vi "insertHTBinData1.vi"(8 "error in (no error)":errorcluster, 9 "FileName":string, 10 "String":string, 11 "connection reference":T2) -> (0 "error out":errorcluster, 1 "concatenated string":string, 3 "connection reference out":T2)   [LabVIEW 2012]
uses:
  <vilib>/addons/database/Connection.llb/Conn ObjectReference.ctl
  <vilib>/addons/database/NI_Database_API.lvlib
panel:
  out "output cluster 2":T1
  out "String 4":string
  out "String 3":string
  out "String 2":string
  out "substring 4":string
  out "before substring":string
  out "substring 3":string
  out "offset past match":i32
  out "after substring 3":string
  in  "input cluster  2":T1
  out "size(s)":i32
  out "E2":i32
  out "S4":string
  out "S5":string
  out "S6":string
  out "S3":string
  out "S2":string
  out "S1":string
  out "array":string[][](array[string])
  out "String":string
  out "output cluster":T1
  in  "input cluster":T1
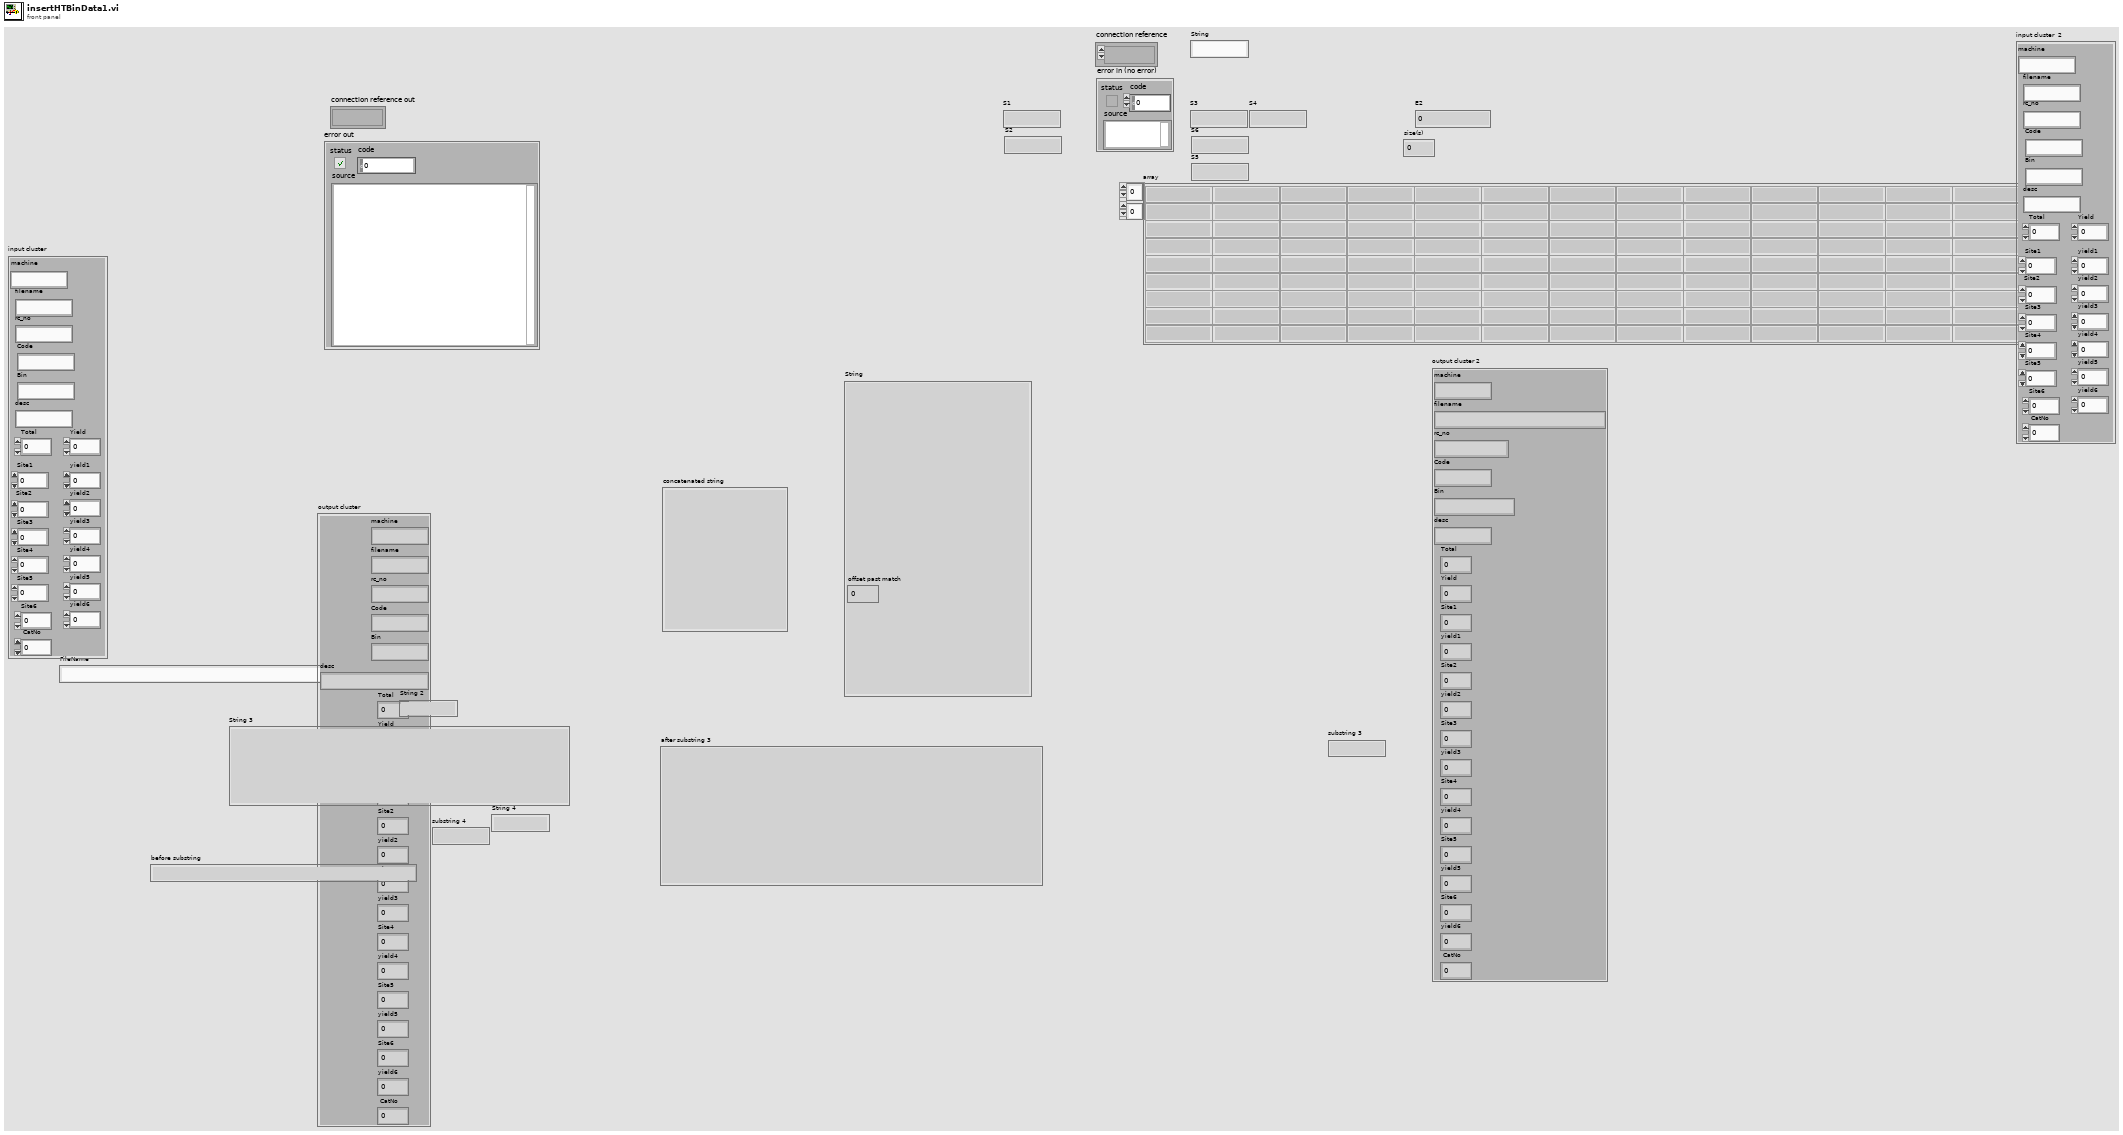
[diagram p1: front panel]
types:
  T1 = cluster{"machine":string, "filename":string, "rc_no":string, "Code":string, "Bin":string, "desc":string, "Total":dbl, "Yield":dbl, "Site1":dbl, "yield1":dbl, "Site2":dbl, "yield2":dbl, "Site3":dbl, "yield3":dbl, "Site4":dbl, "yield4":dbl, "Site5":dbl, "yield5":dbl, "Site6":dbl, "yield6":dbl, " CatNo":dbl}
  T2 = typedef "NI_Database_API.lvlib/Conn ObjectReference.ctl" = refnum<k1>
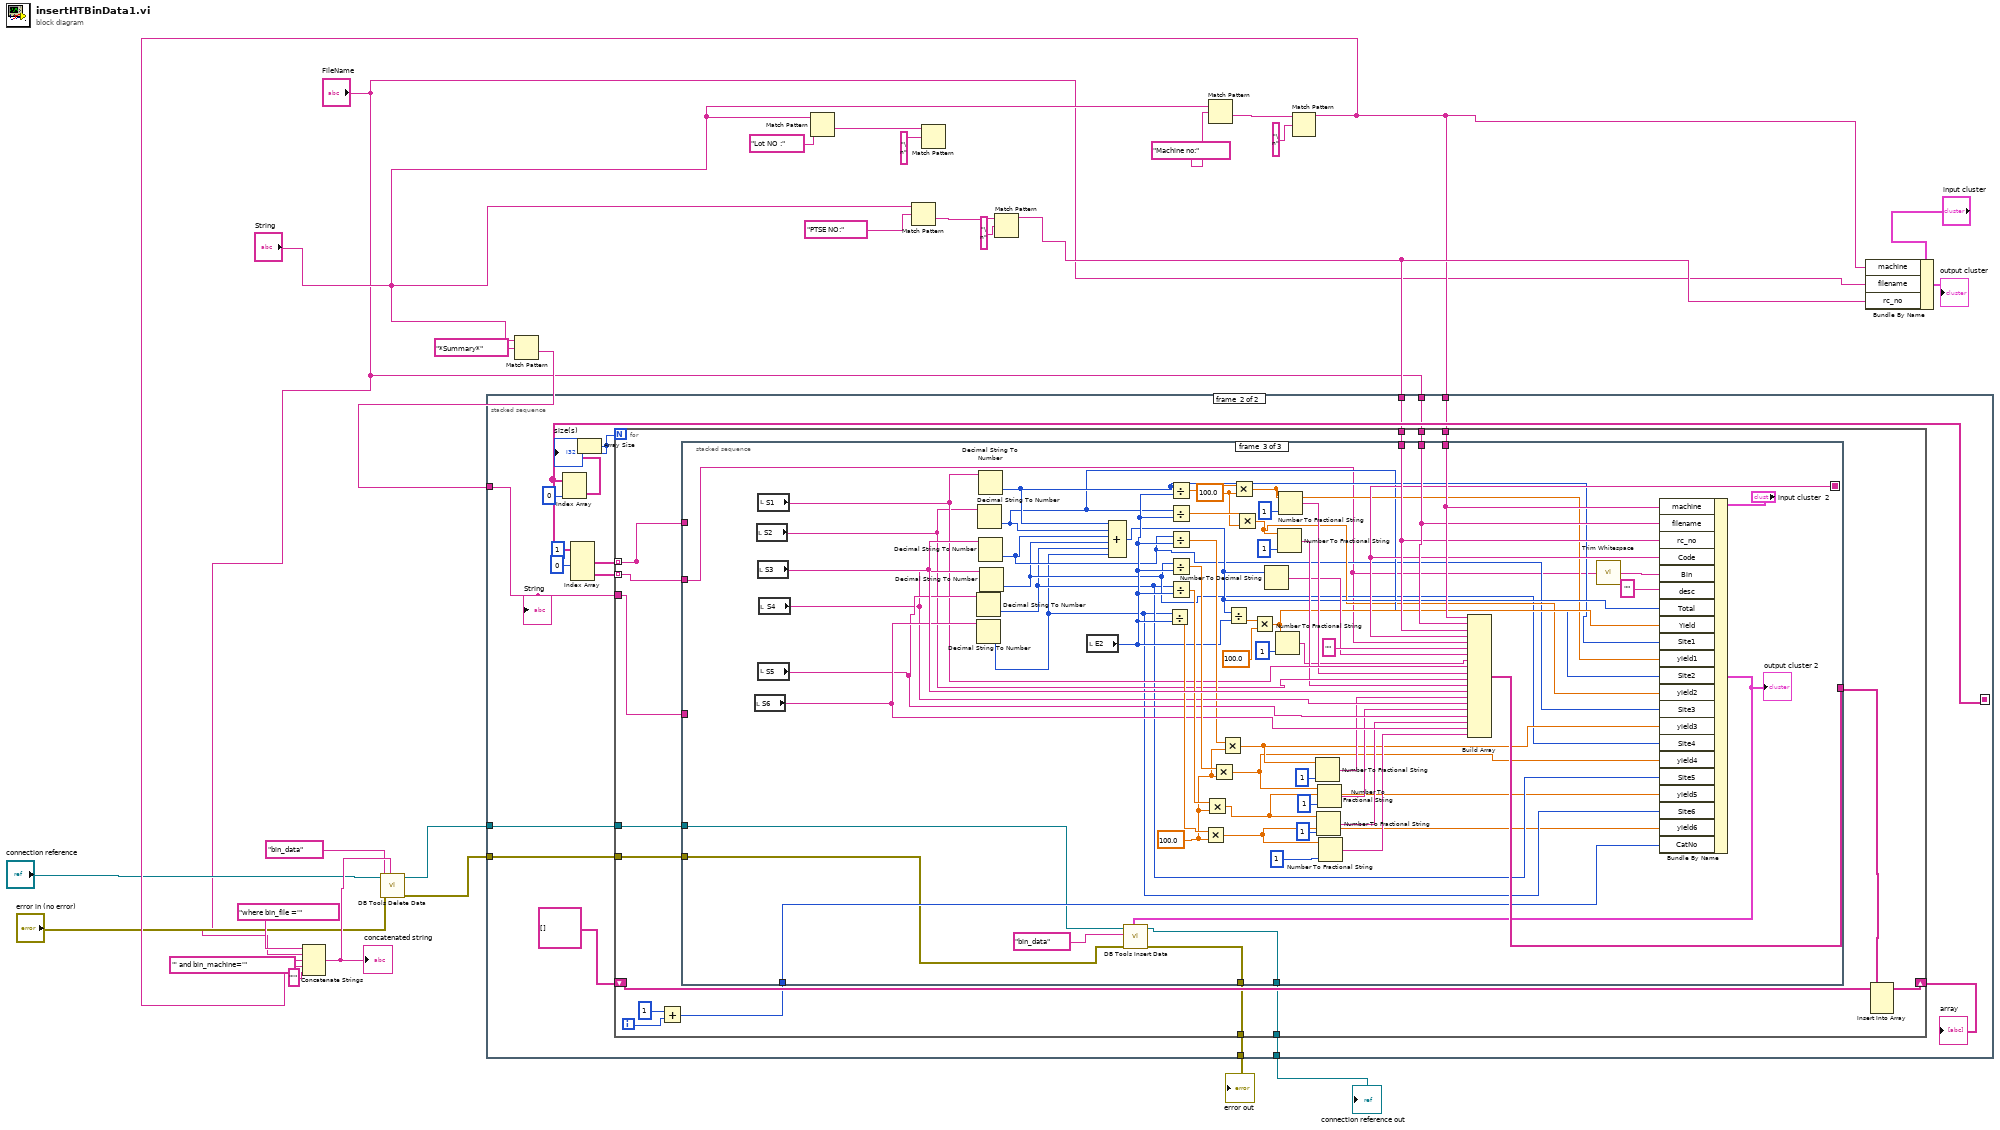
[diagram p0: block diagram]
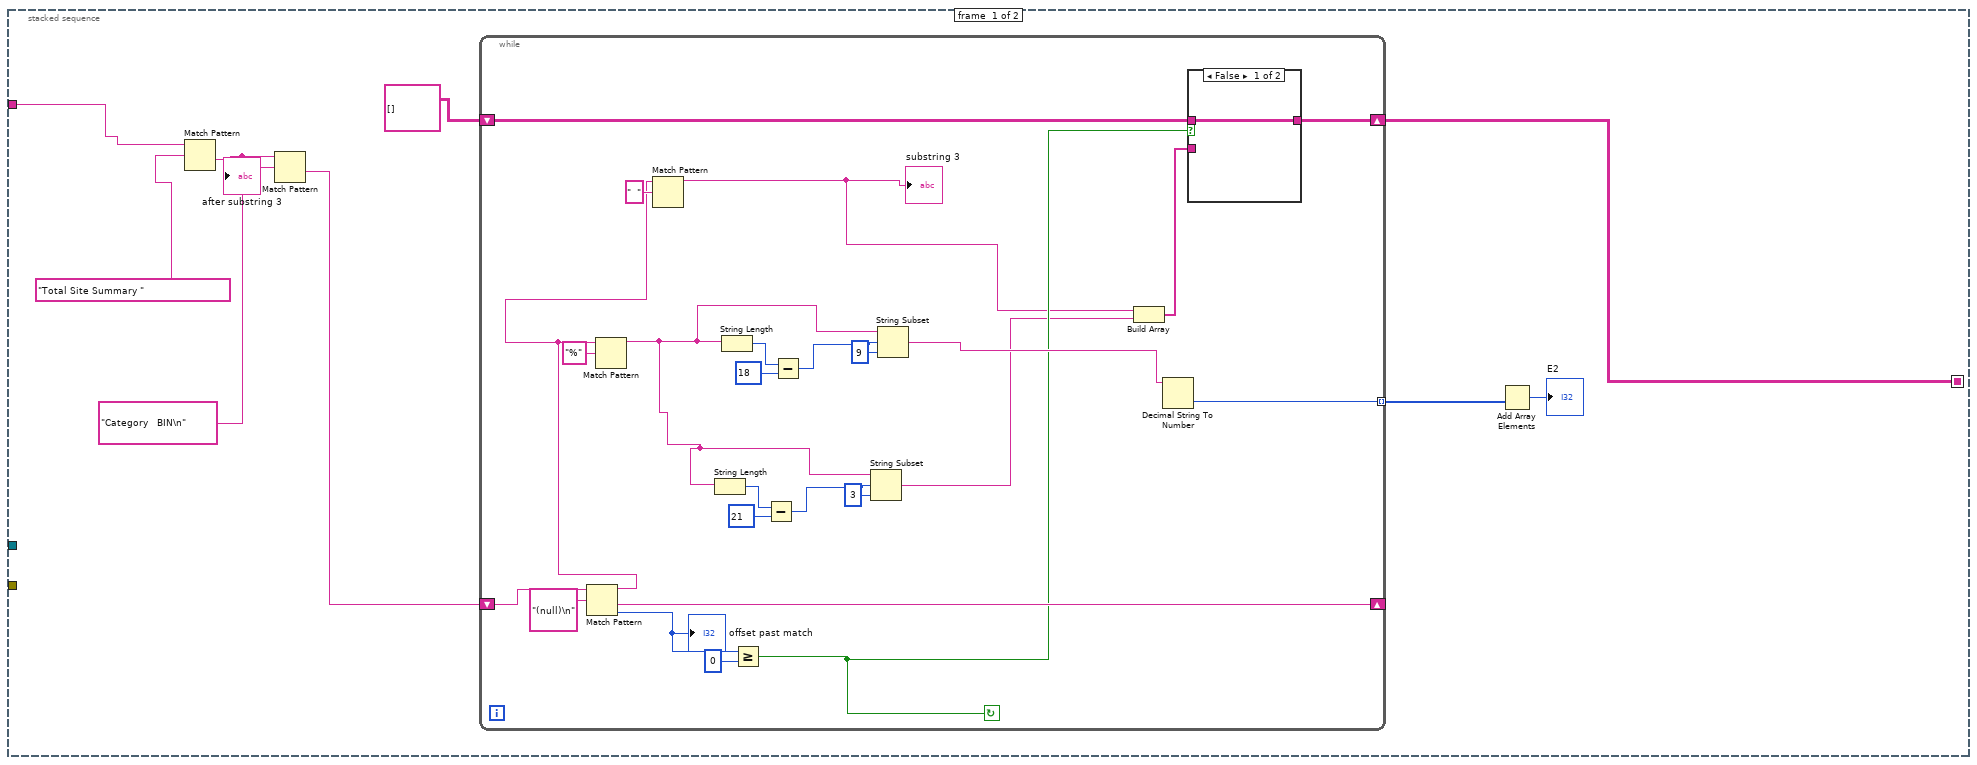
[diagram p2: hidden frame]
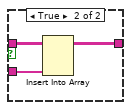
[diagram p3: hidden frame]
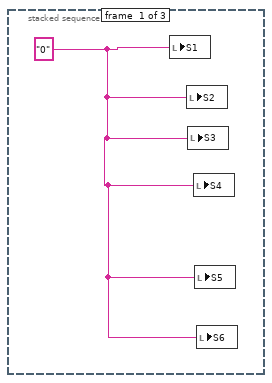
[diagram p4: hidden frame]
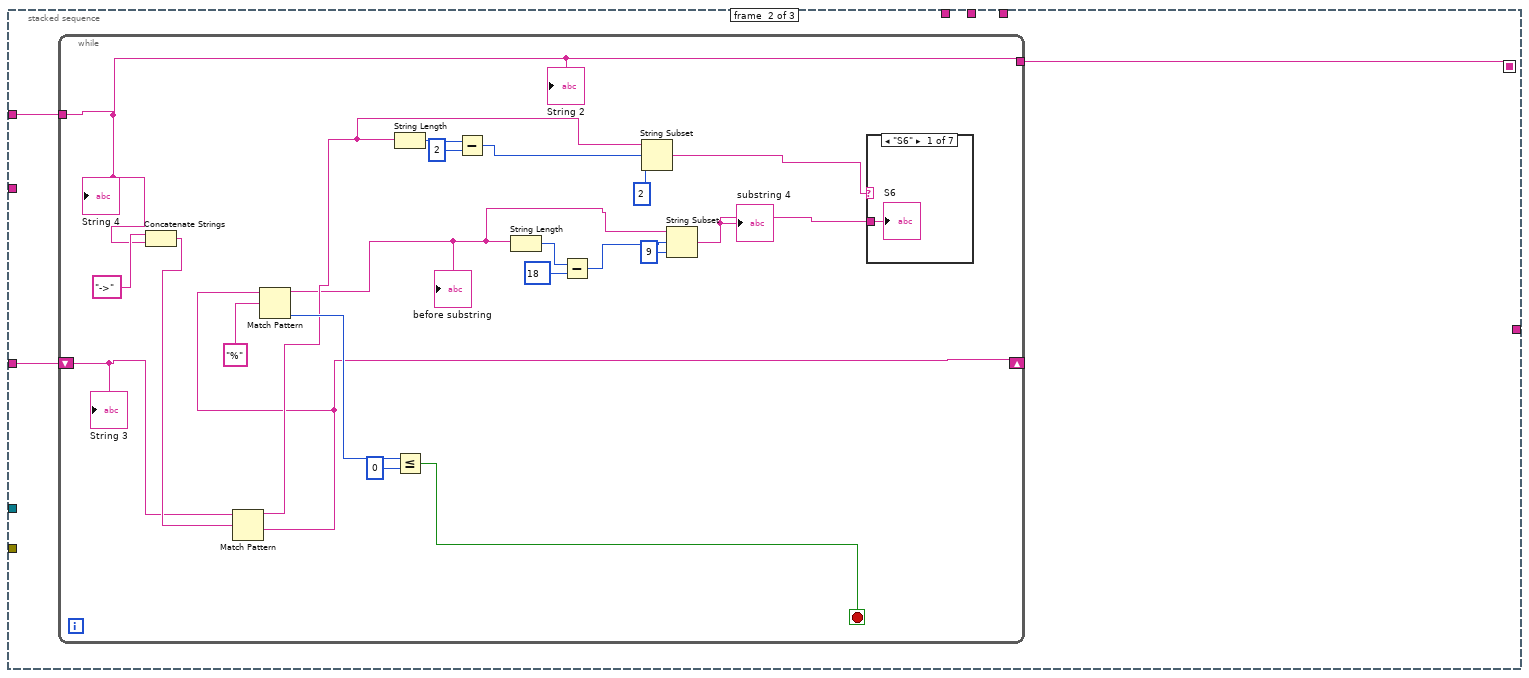
[diagram p5: hidden frame]
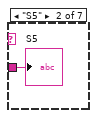
[diagram p6: hidden frame]
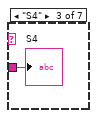
[diagram p7: hidden frame]
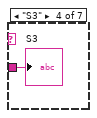
[diagram p8: hidden frame]
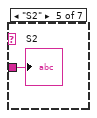
[diagram p9: hidden frame]
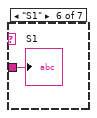
[diagram p10: hidden frame]
diagram:
  n1 = Match Pattern(string="String", regular expression="*Summary*") -> (after substring=w16:string)  [unwired: 1 in, 3 out]
  n2 = Match Pattern(string="String", regular expression="Lot NO :") -> (after substring=w27:string)  [unwired: 1 in, 3 out]
  n3 = Match Pattern(string="String", regular expression="PTSE NO:") -> (after substring=w21:string)  [unwired: 1 in, 3 out]
  n4 = Match Pattern(string=w27, regular expression="\n") -> ()  [unwired: 1 in, 4 out]
  n5 = Match Pattern(string=w21, regular expression="\n") -> (before substring=w15:string)  [unwired: 1 in, 3 out]
  n6 = Match Pattern(string="String", regular expression="Machine no:") -> (after substring=w24:string)  [unwired: 1 in, 3 out]
  n7 = Match Pattern(string=w24, regular expression="\n") -> (before substring=w9:string)  [unwired: 1 in, 3 out]
  n8 = Concatenate Strings("where bin_file ='" ("SQL query"), "FileName", "' and bin_machine='" ("string"), w9, "'" ("string")) -> (w11:string)
  "concatenated string" <- w11
  n9 = call <vilib>:"DB Tools Delete Data.vi"("condition"=w11, "error in (no error)"="error in (no error)", "table"="bin_data", "connection reference"="connection reference") -> ("error out"=w7:errorcluster, "connection reference out"=w8:T2)  [unwired: 6 in]
  n10 = stacked-sequence {
    seq-local: [w29 _] -> [_ w79]
    tunnel: w16 -> [w33 w84]
    tunnel: "FileName" -> [_ w73]
    tunnel: w9 -> [_ w72]
    tunnel: w15 -> [_ w71]
    tunnel: w8 -> [_ w70]
    tunnel: w7 -> [_ w69]
    tunnel: [_ w68] -> w2
    tunnel: [_ w67] -> w1
    frame #0 {
      n11 = Match Pattern(string=w33, regular expression="Total Site Summary ") -> (after substring=w36:string)  [unwired: 1 in, 3 out]
      "after substring 3" <- w36
      n12 = Match Pattern(string=w36, regular expression="Category   BIN\n") -> (after substring=w31:string)  [unwired: 1 in, 3 out]
      n13 = while {
        shift-right: [w50] -> _
        shift-left: w31 -> [w49]
        tunnel: [w44] -> w30 mode=indexing
        shift-right: [w42] -> w29
        shift-left: string[][] [] ("array") -> [w41]
        stop <- w40 continue-if-true
        n14 = Match Pattern(string=w49, regular expression="(null)\n") -> (before substring=w46:string, after substring=w50:string, offset past match=w48:i32)  [unwired: 1 in, 1 out]
        "offset past match" <- w48
        n15 = Match Pattern(string=w46, regular expression="%") -> (before substring=w53:string)  [unwired: 1 in, 3 out]
        n16 = Match Pattern(string=w46, regular expression="  ") -> (before substring=w39:string)  [unwired: 1 in, 3 out]
        "substring 3" <- w39
        n17 = String Length(string=w53) -> (length=w57:i32)
        n18 = String Length(string=w53) -> (length=w61:i32)
        n19 = Greater Or Equal?(x=w48, y=0) -> (x >= y?=w40:bool)
        n20 = Subtract(x=w57, y=21) -> (x-y=w55:i32)
        n21 = Subtract(x=w61, y=18) -> (x-y=w59:i32)
        n22 = String Subset(string=w53, offset (0)=w55, length (rest)=3 ("length (rest)")) -> (substring=w38:string)
        n23 = String Subset(string=w53, offset (0)=w59, length (rest)=9 ("length (rest)")) -> (substring=w45:string)
        n24 = Build Array(w39, w38) -> (w43:string[])
        n25 = Decimal String To Number(string=w45) -> (number=w44:i32)  [unwired: 2 in, 1 out]
        n26 = case shown="False" w40 {
          tunnel: w43 -> [_ w66]
          tunnel: [w63 w65] -> w42
          tunnel: w41 -> [w63 w64]
          frame False {
          }
          frame True {
            n27 = Insert Into Array(array=w64, new element=w66) -> (w65:string[][])  [unwired: 2 in]
          }
        }
      }
      n28 = Add Array Elements(numeric array=w30) -> (sum=→"E2":i32)
    }
    frame #1 {
      n29 = Index Array(array=w79, index (col)=0 ("disabled index (col)")) -> (element=w80:string[])  [unwired: 1 in]
      n30 = Index Array(array=w79, index (col) #1=0 ("disabled index (col)"), index (col) #2=1 ("index (col)")) -> (element #1=w76:string[], element #2=w74:string[])  [unwired: 2 in]
      n31 = Array Size(array=w80) -> (size(s)=w81:i32)
      "size(s)" <- w81
      n32 = for {
        N: w81 -> [_]
        tunnel: w84 -> [w100]
        shift-right: [w99] -> w82
        shift-left: string[][] [] ("array") -> [w98]
        tunnel: [w96] -> _ mode=indexing
        tunnel: w76 -> [w96] mode=indexing
        tunnel: w74 -> [w95] mode=indexing
        tunnel: w73 -> [w94]
        tunnel: w72 -> [w93]
        tunnel: w71 -> [w92]
        tunnel: w70 -> [w88]
        tunnel: w69 -> [w87]
        tunnel: [w86] -> w68
        tunnel: [w85] -> w67
        i -> [w91]
        n33 = Add(x=1, y=w91) -> (x+y=w89:i32)
        n34 = stacked-sequence {
          seq-local: [_ w102 _] -> [_ _ w156]
          tunnel: w100 -> [_ w104 _]
          tunnel: w96 -> [_ w103 _]
          tunnel: [_ _ w194] -> w97
          tunnel: w95 -> [_ _ w132]
          tunnel: w94 -> [_ _ w158]
          tunnel: w93 -> [_ _ w159]
          tunnel: w92 -> [_ _ w157]
          tunnel: w89 -> [_ _ w140]
          tunnel: w88 -> [_ _ w139]
          tunnel: w87 -> [_ _ w137]
          tunnel: [_ _ w135] -> w86
          tunnel: [_ _ w134] -> w85
          frame #0 {
            w101 = "0" ("S1")
            n35 = local write "S1"(w101) -> ()
            n36 = local write "S2"(w101) -> ()
            n37 = local write "S3"(w101) -> ()
            n38 = local write "S4"(w101) -> ()
            n39 = local write "S5"(w101) -> ()
            n40 = local write "S6"(w101) -> ()
          }
          frame #1 {
            n41 = while {
              tunnel: w103 -> [w110]
              shift-right: [w109] -> _
              shift-left: w104 -> [w107]
              tunnel: [w110] -> w102
              stop <- w108 stop-if-true
              n42 = Concatenate Strings("->" ("string"), w110) -> (w113:string)
              n43 = Match Pattern(string=w107, regular expression=w113) -> (before substring=w112:string, after substring=w109:string)  [unwired: 1 in, 2 out]
              n44 = Match Pattern(string=w109, regular expression="%") -> (before substring=w111:string, offset past match=w118:i32)  [unwired: 1 in, 2 out]
              "before substring" <- w111
              n45 = String Length(string=w112) -> (length=w117:i32)
              n46 = Less Or Equal?(x=w118, y=0) -> (x <= y?=w108:bool)
              n47 = Subtract(x=w117, y=2) -> (x-y=w115:i32)
              n48 = String Length(string=w111) -> (length=w124:i32)
              n49 = Subtract(x=w124, y=18) -> (x-y=w122:i32)
              n50 = String Subset(string=w112, offset (0)=w115, length (rest)=2 ("length (rest)")) -> (substring=w105:string)
              n51 = String Subset(string=w111, offset (0)=w122, length (rest)=9 ("length (rest)")) -> (substring=w106:string)
              "substring 4" <- w106
              n52 = case shown="\"S6\"" w105 {
                tunnel: w106 -> [w126 w127 w128 w129 w130 w131 _]
                frame "S6" {
                  "S6" <- w126
                }
                frame "S5" {
                  "S5" <- w127
                }
                frame "S4" {
                  "S4" <- w128
                }
                frame "S3" {
                  "S3" <- w129
                }
                frame "S2" {
                  "S2" <- w130
                }
                frame "S1" {
                  "S1" <- w131
                }
                frame "E2", Default {
                }
              }
              "String 2" <- w110
              "String 3" <- w107
              "String 4" <- w110
            }
          }
          frame #2 {
            w177 = 100.0 ("y")
            w180 = 100.0 ("y")
            n53 = local read "S6"() -> (w187:string)
            n54 = local read "S2"() -> (w174:string)
            n55 = local read "S3"() -> (w193:string)
            n56 = local read "S1"() -> (w176:string)
            n57 = local read "S5"() -> (w185:string)
            n58 = local read "S4"() -> (w183:string)
            n59 = Decimal String To Number(string=w185) -> (number=w144:i32)  [unwired: 2 in, 1 out]
            n60 = Decimal String To Number(string=w187) -> (number=w142:i32)  [unwired: 2 in, 1 out]
            n61 = Decimal String To Number(string=w174) -> (number=w150:i32)  [unwired: 2 in, 1 out]
            n62 = Decimal String To Number(string=w176) -> (number=w152:i32)  [unwired: 2 in, 1 out]
            n63 = Decimal String To Number(string=w193) -> (number=w148:i32)  [unwired: 2 in, 1 out]
            n64 = Decimal String To Number(string=w183) -> (number=w146:i32)  [unwired: 2 in, 1 out]
            n65 = local read "E2"() -> (w170:i32)
            n66 = Compound Arithmetic op=ADD(w152, w150, w148, w146, w144, w142) -> (w154:i32)
            n67 = Divide(x=w142, y=w170) -> (x/y=w191:dbl)
            n68 = Divide(x=w152, y=w170) -> (x/y=w179:dbl)
            n69 = Divide(x=w150, y=w170) -> (x/y=w178:dbl)
            n70 = Divide(x=w148, y=w170) -> (x/y=w181:dbl)
            n71 = Divide(x=w146, y=w170) -> (x/y=w189:dbl)
            n72 = Divide(x=w144, y=w170) -> (x/y=w190:dbl)
            n73 = Multiply(x=w191, y=w180) -> (x*y=w141:dbl)
            n74 = Multiply(x=w190, y=w180) -> (x*y=w143:dbl)
            n75 = Multiply(x=w189, y=w180) -> (x*y=w145:dbl)
            n76 = Multiply(x=w181, y=w180) -> (x*y=w147:dbl)
            n77 = Divide(x=w154, y=w170) -> (x/y=w169:dbl)
            n78 = Multiply(x=w179, y=w177) -> (x*y=w151:dbl)
            n79 = Multiply(x=w178, y=w177) -> (x*y=w149:dbl)
            n80 = Multiply(x=w169, y=100.0) -> (x*y=w153:dbl)
            n81 = Number To Decimal String(number=w154) -> (decimal integer string=w171:string)  [unwired: 1 in]
            n82 = Number To Fractional String(number=w153, precision (6)=i16 1) -> (F-format string=w167:string)  [unwired: 2 in]
            n83 = Number To Fractional String(number=w149, precision (6)=i16 1) -> (F-format string=w173:string)  [unwired: 2 in]
            n84 = Number To Fractional String(number=w151, precision (6)=i16 1) -> (F-format string=w175:string)  [unwired: 2 in]
            n85 = Number To Fractional String(number=w147, precision (6)=i16 1) -> (F-format string=w182:string)  [unwired: 2 in]
            n86 = Number To Fractional String(number=w143, precision (6)=i16 1) -> (F-format string=w186:string)  [unwired: 2 in]
            n87 = Number To Fractional String(number=w145, precision (6)=i16 1) -> (F-format string=w184:string)  [unwired: 2 in]
            n88 = Number To Fractional String(number=w141, precision (6)=i16 1) -> (F-format string=w188:string)  [unwired: 2 in]
            n89 = Build Array(w159, w158, w157, w156, w132, "" ("element"), w171, w167, w176, w175, w174, w173, w193, w182, w183, w184, w185, w186, w187, w188) -> (w194:string[])
            n90 = call <vilib>:"Trim Whitespace.vi"("string"=w132) -> ("trimmed string"=w133:string)  [unwired: 1 in]
            n91 = Bundle By Name(cluster="input cluster  2", "machine"=w159, "filename"=w158, "rc_no"=w157, "Code"=w156, "Bin"=w133, "desc"="", "Total"=w154, "Yield"=w153, "Site1"=w152, "yield1"=w151, "Site2"=w150, "yield2"=w149, "Site3"=w148, "yield3"=w147, "Site4"=w146, "yield4"=w145, "Site5"=w144, "yield5"=w143, "Site6"=w142, "yield6"=w141, "CatNo"=w140) -> (w136:T1)
            "output cluster 2" <- w136
            n92 = call <vilib>:"DB Tools Insert Data.vi"("data"=w136, "error in (no error)"=w137, "table"="bin_data", "connection reference"=w139) -> ("error out"=w134:errorcluster, "connection reference out"=w135:T2)  [unwired: 6 in]
          }
        }
        n93 = Insert Into Array(array=w98, new element=w97) -> (w99:string[][])  [unwired: 2 in]
      }
      "array" <- w82
      "String" <- w84
    }
  }
  "connection reference out" <- w2
  "error out" <- w1
  n94 = Bundle By Name(cluster="input cluster", "machine"=w9, "filename"="FileName", "rc_no"=w15) -> (→"output cluster":T1)
